vi "Template Get All.vi"(8 "error in (no error)":errorcluster, 10 "Order By (\"sxTemplateId\")":string="sxTemplateId", 11 "Connection Refnum":T1) -> (0 "error out":errorcluster, 2 "Templates":T2[](array[typedef]), 3 "Connection Refnum":T1, 4 "Data Present":bool)   [LabVIEW 2011]
uses:
  Template Record.ctl
  SI.LIB/ODBC/SQL Controls/Connection Refnum.ctl
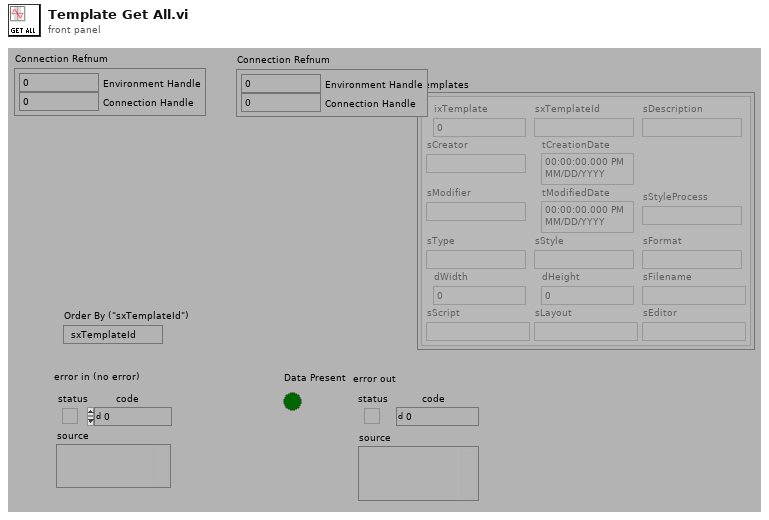
[diagram p1: front panel]
types:
  T1 = typedef "Connection Refnum.ctl" = cluster{"Environment Handle":i32, "Connection Handle":i32}
  T2 = typedef "Template Record.ctl" = cluster{"ixTemplate":i32, "sxTemplateId":string, "sDescription":string, "sCreator":string, "tCreationDate":timestamp, "sModifier":string, "tModifiedDate":timestamp, "sType":string, "sStyle":string, "sFormat":string, "dWidth":dbl, "dHeight":dbl, "sFilename":string, "sScript":string, "sLayout":string, "sEditor":string, "sStyleProcess":string}
  T3 = typedef "Statement Refnum.ctl" = cluster{"Statement Handle":i32, "Parameter Number":u16}
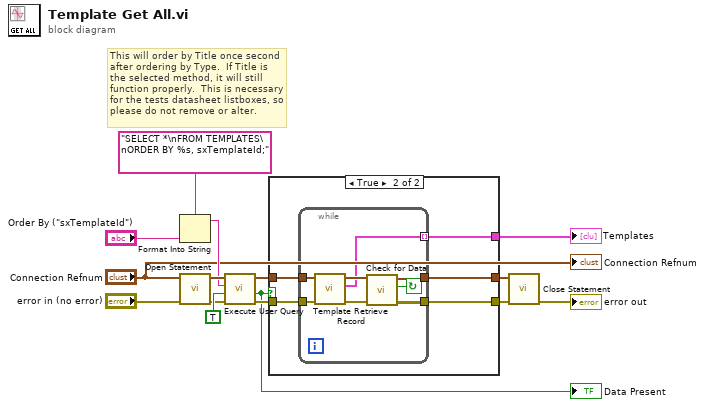
[diagram p0: block diagram]
diagram:
  # "This will order by Title once second\nafter ordering by Type.  If Title is\nthe selected method, it will still \nfunction properly.  This is necessary\nfor the tests datasheet listboxes, so\nplease do not remove or alter."
  n1 = Format Into String(format string="SELECT *\nFROM TEMPLATES\nORDER BY %s, sxTemplateId;" ("Query Name"), "Order By (\"sxTemplateId\")") -> (resulting string=w5:string)  [unwired: 2 in, 1 out]
  n2 = call "Open Statement.vi"("error in (no error)"="error in (no error)", "Connection Refnum"="Connection Refnum") -> ("error out"=w9:errorcluster, "Statement Refnum"=w10:T3)  [unwired: 4 out]
  n3 = call "Execute User Query.vi"("error in (no error)"=w9, "Return Data? (f)"=TRUE, "User Query"=w5, "Statement Refnum"=w10) -> ("error out"=w15:errorcluster, "Data Present?"=w8:bool, "Statement Refnum"=w14:T3)  [unwired: 1 out]
  "Data Present" <- w8
  n4 = case shown="True" w8 {
    tunnel: w15 -> [w16 w21]
    tunnel: w14 -> [w17 w22]
    tunnel: [w16 w19] -> w11
    tunnel: [w17 w20] -> w12
    tunnel: [_ w18] -> w4
    frame False {
    }
    frame True {
      n5 = while {
        tunnel: w22 -> [w29]
        tunnel: w21 -> [w28]
        tunnel: [w26] -> w20
        tunnel: [w24] -> w19
        tunnel: [w23] -> w18 mode=indexing
        stop <- w30 continue-if-true
        n6 = call "Template Retrieve Record.vi"("error in (no error)"=w28, "Statement Refnum"=w29) -> ("error out"=w25:errorcluster, "Template Record"=w23:T2, "Statement Refnum"=w27:T3)  [unwired: 7 out]
        n7 = call "Check for Data.vi"("error in (no error)"=w25, "Statement Refnum"=w27) -> ("error out"=w24:errorcluster, "Data Present?"=w30:bool, "Statement Refnum"=w26:T3)  [unwired: 3 out]
      }
    }
  }
  "Templates" <- w4
  n8 = call "Close Statement.vi"("error in (no error)"=w11, "Statement Refnum"=w12) -> ("error out"=→"error out":errorcluster)  [unwired: 5 out]
  "Connection Refnum" <- "Connection Refnum"
